vi "WristTeleop.vi"(3 "Floor":bool, 4 "Source":bool, 6 "Rest":bool, 7 "Cancel":bool, 8 "Slant":bool, 9 "Flat":bool, 10 "Dec":bool, 11 "Inc":bool) -> ()   [LabVIEW 2023]
doc: "Controls Wrist positions. If corresponding Boolean inputs are True, then case structure becomes True which calls SendCmds for various Wrist positions. Inc and Dec can be held down, the rest are OnEdge as they are setpoints.\n\nInputs:\n--Cancel--Boolean--(cancels wrist demands)\n--Inc--Boolean--incrementor (wrist angle up)\n--Dec--Boolean--decrenentor (wrist angle down)\n--Flat--Boolean--setpoint (0 deg, L1-L3)\n--Slant--Boolean--setpoint (-36 deg, L4)\n--Rest--Boolean--setpoint (-90, inside perim)"
uses:
  <vilib>/Rock Robotics/WPI/ThirdParty/JAS_Junk/TrajLib/VI/BoolCmd_Send.vi
  <vilib>/Rock Robotics/WPI/ThirdParty/JAS_Junk/TrajLib/VI/BoolCmd_Send_Internal.vi
  <vilib>/Rock Robotics/WPI/ThirdParty/JAS_Junk/TrajLib/VI/BoolCmd_ObtainQueue.vi
  <vilib>/Rock Robotics/WPI/ThirdParty/JAS_Junk/TrajLib/Trajectory_Library.lvlib
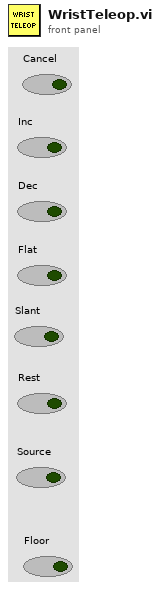
[diagram p1: front panel]
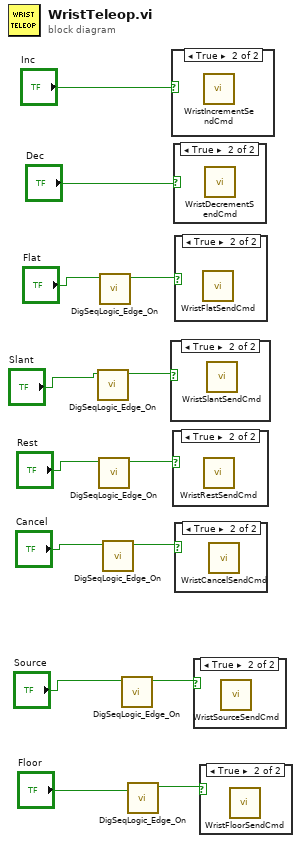
[diagram p0: block diagram]
diagram:
  n1 = call <vilib>:"DigSeqLogic_Edge_On.vi"("Input"="Slant") -> ("On Edge"=w11:bool)  [unwired: 10 in]
  n2 = call <vilib>:"DigSeqLogic_Edge_On.vi"("Input"="Rest") -> ("On Edge"=w12:bool)  [unwired: 10 in]
  n3 = call <vilib>:"DigSeqLogic_Edge_On.vi"("Input"="Flat") -> ("On Edge"=w14:bool)  [unwired: 10 in]
  n4 = call <vilib>:"DigSeqLogic_Edge_On.vi"("Input"="Cancel") -> ("On Edge"=w13:bool)  [unwired: 10 in]
  n5 = call <vilib>:"DigSeqLogic_Edge_On.vi"("Input"="Source") -> ("On Edge"=w4:bool)  [unwired: 10 in]
  n6 = call <vilib>:"DigSeqLogic_Edge_On.vi"("Input"="Floor") -> ("On Edge"=w2:bool)  [unwired: 10 in]
  n7 = case shown="True" w11 {
    frame False {
    }
    frame True {
      n8 = call "WristSlantSendCmd.vi"() -> ()  [unwired: 11 in, 1 out]
    }
  }
  n9 = case shown="True" "Inc" {
    frame False {
    }
    frame True {
      n10 = call "WristIncrementSendCmd.vi"() -> ()  [unwired: 11 in, 1 out]
    }
  }
  n11 = case shown="True" w12 {
    frame False {
    }
    frame True {
      n12 = call "WristRestSendCmd.vi"() -> ()  [unwired: 11 in, 1 out]
    }
  }
  n13 = case shown="True" "Dec" {
    frame False {
    }
    frame True {
      n14 = call "WristDecrementSendCmd.vi"() -> ()  [unwired: 11 in, 1 out]
    }
  }
  n15 = case shown="True" w14 {
    frame False {
    }
    frame True {
      n16 = call "WristFlatSendCmd.vi"() -> ()  [unwired: 11 in, 1 out]
    }
  }
  n17 = case shown="True" w13 {
    frame False {
    }
    frame True {
      n18 = call "WristCancelSendCmd.vi"() -> ()  [unwired: 11 in, 1 out]
    }
  }
  n19 = case shown="True" w4 {
    frame False {
    }
    frame True {
      n20 = call "WristSourceSendCmd.vi"() -> ()  [unwired: 11 in, 1 out]
    }
  }
  n21 = case shown="True" w2 {
    frame False {
    }
    frame True {
      n22 = call "WristFloorSendCmd.vi"() -> ()  [unwired: 11 in, 1 out]
    }
  }
